vi "TDC_DAQV14_after_500MHz.vi"() -> ()   [LabVIEW 2017]
uses:
  <vilib>/Utility/file.llb/Write Delimited Spreadsheet (DBL).vi
  <vilib>/Utility/file.llb/Write Delimited Spreadsheet (I64).vi
panel:
  out "data out":string
  in  "display":bool
  in  "Thresholds":u16
  in  "one key for threshold":bool
  in  "save data":bool=TRUE
  in  "RST":bool
  out "rate":dbl=24091.155888084242
  in  "Thresholds (mV)":u16[](array[numeric])=[500, 500, 500, 500, 500, 500, 500, 500]
  out "appended path 2":path=path "G:/tdc/2017/test_20230331_123130.csv"
  in  "通道数量":i32=64
  out "Cal Table":u32[](array[numeric])=[100002, 100002, 100002, 100002, 100002, 100002, 100002, 100002, 100002, 100002, 100002, 100002, 100002, 100002, 100002, 100002, 100002, 100002, 100002, 100002, 100002, 100002, 100002, 100002, 100002, 100002, 100002, 100002, 100002, 100002, 100002, 100002, 100002, 100002, 100002, 100002, 100002, 100002, 100002, 100002, 100002, 100002, 100002, 100002, 100002, 100002, 100002, 100002, 100002, 100002, 100002, 100002, 100002, 100002, 100002, 100002, 100002, 100002, 100002, 100002, 100002, 100002, 100002, 100002]
  in  "channel for cal":i32=41
  out "single":u32 format="%08x"
  out "channel number":u64
  in  "bytes to read":i32=80
  out "Calibration Counter":i32=100000
  out "Event index":i32=97959
  out "cal":u32[](graph)=[0, 0, 0, 0, 0, 0, 0, 0, 0, 0, 0, 0, 0, 0, 0, 0, 0, 0, 0, 0, 0, 0, 0, 0, 0, 0, 0, 0, 0, 0, 0, 0, 0, 0, 0, 0, 0, 0, 0, 0, 0, 0, 0, 0, 0, 0, 0, 0, 0, 0, 0, 0, 0, 0, 0, 0, 0, 0, 0, 0, 0, 0, 0, 0, 0, 0, 0, 0, 0, 0, 0, 0, 0, 0, 0, 0, 0, 0, 0, 0, 0, 0, 0, 0, 0, 0, 0, 0, 0, 0, 0, 0, 0, 0, 0, 0, 0, 0, 0, 0, 0, 0, 0, 0, 0, 0, 0, 0, 0, 0, 0, 0, 0, 0, 0, 0, 0, 0, 0, 0, 0, 0, 0, 0, 0, 0, 0, 0, 0, 0, 0, 0, 0, 0, 0, 0, 0, 0, 0, 0, 0, 0, 0, 0, 0, 0, 0, 0, 0, 0, 0, 0, 0, 0, 0, 0, 0, 0, 0, 0, 0, 0, 0, 0, 0, 0, 0, 0, 0, 0, 0, 0, 0, 0, 0, 0, 0, 0, 0, 0, 0, 0, 0, 0, 0, 0, 0, 0, 0, 0, 0, 0, 0, 0, 0, 0, 0, 0, 0, 0, 0, 0, 0, 0, 0, 0, 0, 0, 0, 0, 0, 0, 0, 0, 0, 0, 0, 0, 0, 0, 0, 0, 0, 0, 0, 0, 0, 0, 0, 0, 0, 0, 0, 0, 0, 0, 0, 0, 0, 0, 0, 0, 0, 0, 0, 0, 0, 0, 0, 0, 0, 0, 0, 0, 0, 0, 0, 0, 0, 0, 0, 0, 0, 0, 0, 0, 0, 0, 0, 0, 0, 0, 0, 0, 0, 0, 0, 0, 0, 0, 0, 0, 0, 0, 69, 70, 200, 130, 69, 246, 200, 570, 155, 125, 160, 737, 265, 234, 80, 72, 155, 352, 178, 160, 101, 206, 84, 365, 186, 117, 86, 60, 156, 209, 124, 214, 202, 261, 117, 73, 308, 242, 175, 128, 73, 81, 167, 174, 75, 216, 363, 315, 84, 97, 67, 59, 109, 150, 167, 160, 255, 179, 72, 87, 290, 76, 119, 326, 114, 45, 62, 78, 150, 147, 151, 162, 202, 176, 82, 116, 138, 114, 75, 113, 110, 101, 122, 201, 217, 141, 136, 157, 107, 58, 72, 121, 214, 134, 190, 85, 127, 40, 49, 167, 84, 94, 55, 140, 150, 323, 144, 120, 198, 82, 104, 145, 98, 145, 124, 102, 120, 122, 116, 182, 125, 271, 123, 141, 162, 133, 69, 215, 207, 175, 168, 104, 108, 78, 53, 79, 151, 49, 89, 85, 85, 111, 122, 183, 115, 76, 52, 103, 55, 195, 80, 148, 66, 203, 83, 109, 86, 127, 131, 146, 160, 56, 237, 116, 94, 113, 99, 196, 68, 98, 110, 100, 172, 79, 169, 116, 117, 123, 110, 65, 74, 191, 201, 60, 82, 145, 203, 331, 56, 81, 133, 70, 159, 77, 112, 99, 387, 124, 150, 144, 130, 139, 195, 199, 128, 218, 147, 185, 205, 192, 146, 108, 97, 131, 101, 111, 84, 118, 163, 85, 177, 88, 182, 180, 61, 157, 82, 351, 115, 106, 74, 143, 109, 258, 313, 81, 165, 89, 58, 85, 204, 137, 246, 384, 77, 54, 56, 35, 35, 56, 80, 104, 166, 240, 104, 141, 174, 99, 41, 45, 48, 342, 180, 52, 34, 51, 82, 107, 274, 80, 228, 263, 129, 87, 73, 132, 104, 176, 471, 227, 175, 92, 123, 87, 132, 208, 250, 311, 62, 78, 114, 117, 138, 66, 205, 68, 65, 77, 89, 222, 101, 35, 32, 93, 426, 159, 207, 108, 118, 397, 204, 160, 183, 94, 81, 319, 221, 353, 107, 148, 53, 77, 134, 155, 112, 111, 231, 165, 106, 57, 49, 105, 122, 283, 91, 135, 227, 130, 44, 139, 101, 136, 222, 141, 96, 146, 191, 123, 61, 106, 123, 177, 186, 188, 104, 123, 156, 140, 100, 64, 374, 103, 60, 168, 144, 148, 130, 95, 162, 194, 107, 167, 74, 45, 67, 215, 229, 107, 63, 222, 202, 123, 240, 160, 148, 120, 139, 175, 82, 103, 141, 143, 202, 174, 62, 150, 156, 284, 140, 86, 136, 150, 198, 220, 264, 88, 56, 69, 65, 69, 85, 66, 84, 107, 133, 510, 177, 52, 53, 55, 110, 95, 96, 83, 124, 150, 123, 178, 95, 62, 75, 88, 69, 95, 35, 50, 75, 183, 97, 251, 162, 179, 180, 93, 65, 169, 112, 116, 177, 208, 184, 68, 75, 142, 98, 71, 150, 172, 202, 395, 214, 117, 49, 50, 82, 91, 115, 199, 198, 93, 89, 64, 109, 107, 126, 100, 146, 150, 289, 93, 85, 109, 265, 257, 120, 105, 81, 143, 123, 142, 119, 95, 119, 215, 82, 168, 280, 111, 80, 82, 356, 76, 69, 92, 169, 83, 86, 299, 88, 276, 65, 78, 63, 82, 83, 177, 100, 201, 200, 190, 121, 241, 193, 119, 52, 71, 41, 83, 299, 57, 49, 89, 383, 57, 104, 116, 97, 125, 140, 90, 500, 118, 131, 99, 266, 88, 120, 136, 137, 67, 284, 70, 104, 197, 134, 97, 65, 58, 91, 59, 60, 151, 249, 196, 119, 123, 237, 171, 123, 194, 186, 327, 72, 73, 99, 109, 71, 77, 83, 280, 299, 156, 122, 105, 70, 71, 57, 69, 134, 243, 113, 44, 98, 115, 59, 69, 95, 101, 71, 91, 99, 174, 162, 58, 64, 63, 516, 81, 69, 57, 41, 74, 56, 81, 52, 102, 98, 117, 102, 214, 291, 137, 66, 67, 101, 69, 93, 95, 166, 66, 117, 262, 138, 91, 82, 112, 120, 164, 98, 141, 218, 129, 81, 149, 194, 418, 79, 63, 79, 143, 157, 171, 123, 164, 295, 81, 83, 71, 229, 94, 291, 240, 117, 169, 63, 155, 82, 115, 184, 82, 120, 90, 124, 256, 88, 117, 146, 38, 47, 368, 150, 86, 26, 89, 131, 94, 175, 84, 175, 206, 184, 110, 89, 134, 125, 258, 82, 248, 85, 82, 183, 85, 284, 160, 108, 55, 60, 137, 59, 58, 105, 136, 68, 51, 58, 290, 461, 126, 83, 52, 150, 63, 27, 40, 19, 10, 2, 0, 0, 0, 0, 0, 0, 0, 0, 0, 0, 0, 0, 0, 0, 0, 0, 0, 0, 0, 0, 0, 0, 0, 0, 0, 0, 0, 0, 0, 0, 0, 0, 0, 0, 0, 0, 0, 0, 0, 0, 0, 0, 0, 0, 0, 0, 0, 0, 0, 0, 0, 0, 0, 0, 0, 0, 0, 0, 0, 0, 0, 0, 0, 0, 0, 0, 0, 0, 0, 0, 0, 0, 0, 0, 0, 0, 0, 0, 0, 0, 0, 0, 0, 0, 0, 0, 0, 0, 0, 0, 0, 0, 0, 0, 0, 0, 0, 0, 0, 0, 0, 0, 0, 0, 0, 0, 0, 0, 0, 0, 0, 0, 0, 0, 0, 0, 0, 0, 0, 0, 0, 0, 0, 0, 0, 0, 0, 0, 0, 0, 0, 0, 0, 0, 0, 0, 0, 0, 0, 0, 0, 0, 0, 0, 0, 0, 0, 0, 0, 0, 0, 0, 0, 0, 0, 0, 0, 0, 0, 0, 0, 0, 0, 0, 0, 0, 0, 0, 0, 0, 0, 0, 0, 0, 0, 0, 0, 0, 0, 0, 0, 0, 0, 0, 0, 0, 0, 0, 0, 0, 0, 0, 0, 0, 0, 0, 0, 0, 0, 0, 0, 0, 0, 0, 0, 0, 0, 0, 0, 0, 0, 0, 0, 0, 0, 0, 0, 0, 0, 0, 0, 0, 0, 0, 0, 0, 0, 0, 0, 0, 0, 0, 0, 0, 0, 0, 0, 0, 0, 0, 0, 0, 0, 0, 0, 0, 0, 0, 0, 0, 0, 0, 0, 0, 0, 0, 0, 0, 0, 0, 0, 0, 0, 0, 0, 0, 0, 0, 0, 0, 0, 0, 0, 0, 0, 0, 0, 0, 0, 0, 0, 0, 0, 0, 0, 0, 0, 0, 0, 0, 0, 0, 0, 0, 0, 0, 0, 0, 0, 0, 0, 0, 0, 0, 0, 0, 0, 0, 0, 0, 0, 0, 0, 0, 0, 0, 0, 0, 0, 0, 0, 0, 0, 0, 0, 0, 0, 0, 0, 0, 0, 0, 0, 0, 0, 0, 0, 0, 0, 0, 0, 0, 0, 0, 0, 0, 0, 0, 0, 0, 0, 0, 0, 0, 0, 0, 0, 0, 0, 0, 0, 0, 0, 0, 0, 0, 0, 0, 0, 0, 0, 0, 0, 0, 0, 0, 0, 0, 0, 0, 0, 0, 0, 0, 0, 0, 0, 0, 0, 0, 0, 0, 0, 0, 0, 0, 0, 0, 0, 0, 0, 0, 0, 0, 0, 0, 0, 0, 0, 0, 0, 0, 0, 0, 0, 0, 0, 0, 0, 0, 0, 0, 0, 0, 0, 0, 0, 0, 0, 0, 0, 0, 0, 0, 0, 0, 0, 0, 0, 0, 0, 0, 0, 0, 0, 0, 0, 0, 0, 0, 0, 0, 0, 0, 0, 0, 0, 0, 0, 0, 0, 0, 0, 0, 0, 0, 0, 0, 0, 0, 0, 0, 0, 0, 0, 0, 0, 0, 0, 0, 0, 0, 0, 0, 0, 0, 0, 0, 0, 0, 0, 0, 0, 0, 0, 0, 0, 0, 0, 0, 0, 0, 0, 0, 0, 0, 0, 0, 0, 0, 0, 0, 0, 0, 0, 0, 0, 0, 0, 0, 0, 0, 0, 0, 0, 0, 0, 0, 0, 0, 0, 0, 0, 0, 0, 0, 0, 0, 0, 0, 0, 0, 0, 0, 0, 0, 0, 0, 0, 0, 0, 0, 0, 0, 0, 0, 0, 0, 0, 0, 0, 0, 0, 0, 0, 0, 0, 0, 0, 0, 0, 0, 0, 0, 0, 0, 0, 0, 0, 0, 0, 0, 0, 0, 0, 0, 0, 0, 0, 0, 0, 0, 0, 0, 0, 0, 0, 0, 0, 0, 0, 0, 0, 0, 0, 0, 0, 0, 0, 0, 0, 0, 0, 0, 0, 0, 0, 0, 0, 0, 0, 0, 0, 0, 0, 0, 0, 0, 0, 0, 0, 0, 0, 0, 0, 0, 0, 0, 0, 0, 0, 0, 0, 0, 0, 0, 0, 0, 0, 0, 0, 0, 0, 0, 0, 0, 0, 0, 0, 0, 0, 0, 0, 0, 0, 0, 0, 0, 0, 0, 0, 0, 0, 0, 0, 0, 0, 0, 0, 0, 0, 0, 0, 0, 0, 0, 0, 0, 0, 0, 0, 0, 0, 0, 0, 0, 0, 0, 0, 0, 0, 0, 0, 0, 0, 0, 0, 0, 0, 0, 0, 0, 0, 0, 0, 0, 0, 0, 0, 0, 0, 0, 0, 0, 0, 0, 0, 0, 0, 0, 0, 0, 0, 0, 0, 0, 0, 0, 0, 0, 0, 0, 0, 0, 0, 0, 0, 0, 0, 0, 0, 0, 0, 0, 0, 0, 0, 0, 0, 0, 0, 0, 0, 0, 0, 0, 0, 0, 0, 0, 0, 0, 0, 0, 0, 0, 0, 0, 0, 0, 0, 0, 0, 0, 0, 0, 0, 0, 0, 0, 0, 0, 0, 0, 0, 0, 0, 0, 0, 0, 0, 0, 0, 0, 0, 0, 0, 0, 0, 0, 0, 0, 0, 0, 0, 0, 0, 0, 0, 0, 0, 0, 0, 0, 0, 0, 0, 0, 0, 0, 0, 0, 0, 0, 0, 0, 0, 0, 0, 0, 0, 0, 0, 0, 0, 0, 0, 0, 0, 0, 0, 0, 0, 0, 0, 0, 0, 0, 0, 0, 0, 0, 0, 0, 0, 0, 0, 0, 0, 0, 0, 0, 0, 0, 0, 0, 0, 0, 0, 0, 0, 0, 0, 0, 0, 0, 0, 0, 0, 0, 0, 0, 0, 0, 0, 0, 0, 0, 0, 0, 0, 0, 0, 0, 0, 0, 0, 0, 0, 0, 0, 0, 0, 0, 0, 0, 0, 0, 0, 0, 0, 0, 0, 0, 0, 0, 0, 0, 0, 0, 0, 0, 0, 0, 0, 0, 0, 0, 0, 0, 0, 0, 0, 0, 0, 0, 0, 0, 0, 0, 0, 0, 0, 0, 0, 0, 0, 0, 0, 0, 0, 0, 0, 0, 0, 0, 0, 0, 0, 0, 0, 0, 0, 0, 0, 0, 0, 0, 0, 0, 0, 0, 0, 0, 0, 0, 0, 0, 0, 0, 0, 0, 0, 0, 0, 0, 0, 0, 0, 0, 0, 0, 0, 0, 0, 0, 0, 0, 0, 0, 0, 0, 0, 0, 0, 0, 0, 0, 0, 0, 0, 0, 0, 0, 0, 0, 0, 0, 0, 0, 0, 0, 0, 0, 0, 0, 0]
  out "error out":errorcluster
  in  "stop":bool=TRUE
  out "appended path":path=path "G:/tdc/2017/test_20230331_123130.dat"
  in  "filename":string="test"
  in  "Events":i32=110000 min=1
  in  "timeout (ms)":i32=10000
  in  "address":string="192.168.10.10"
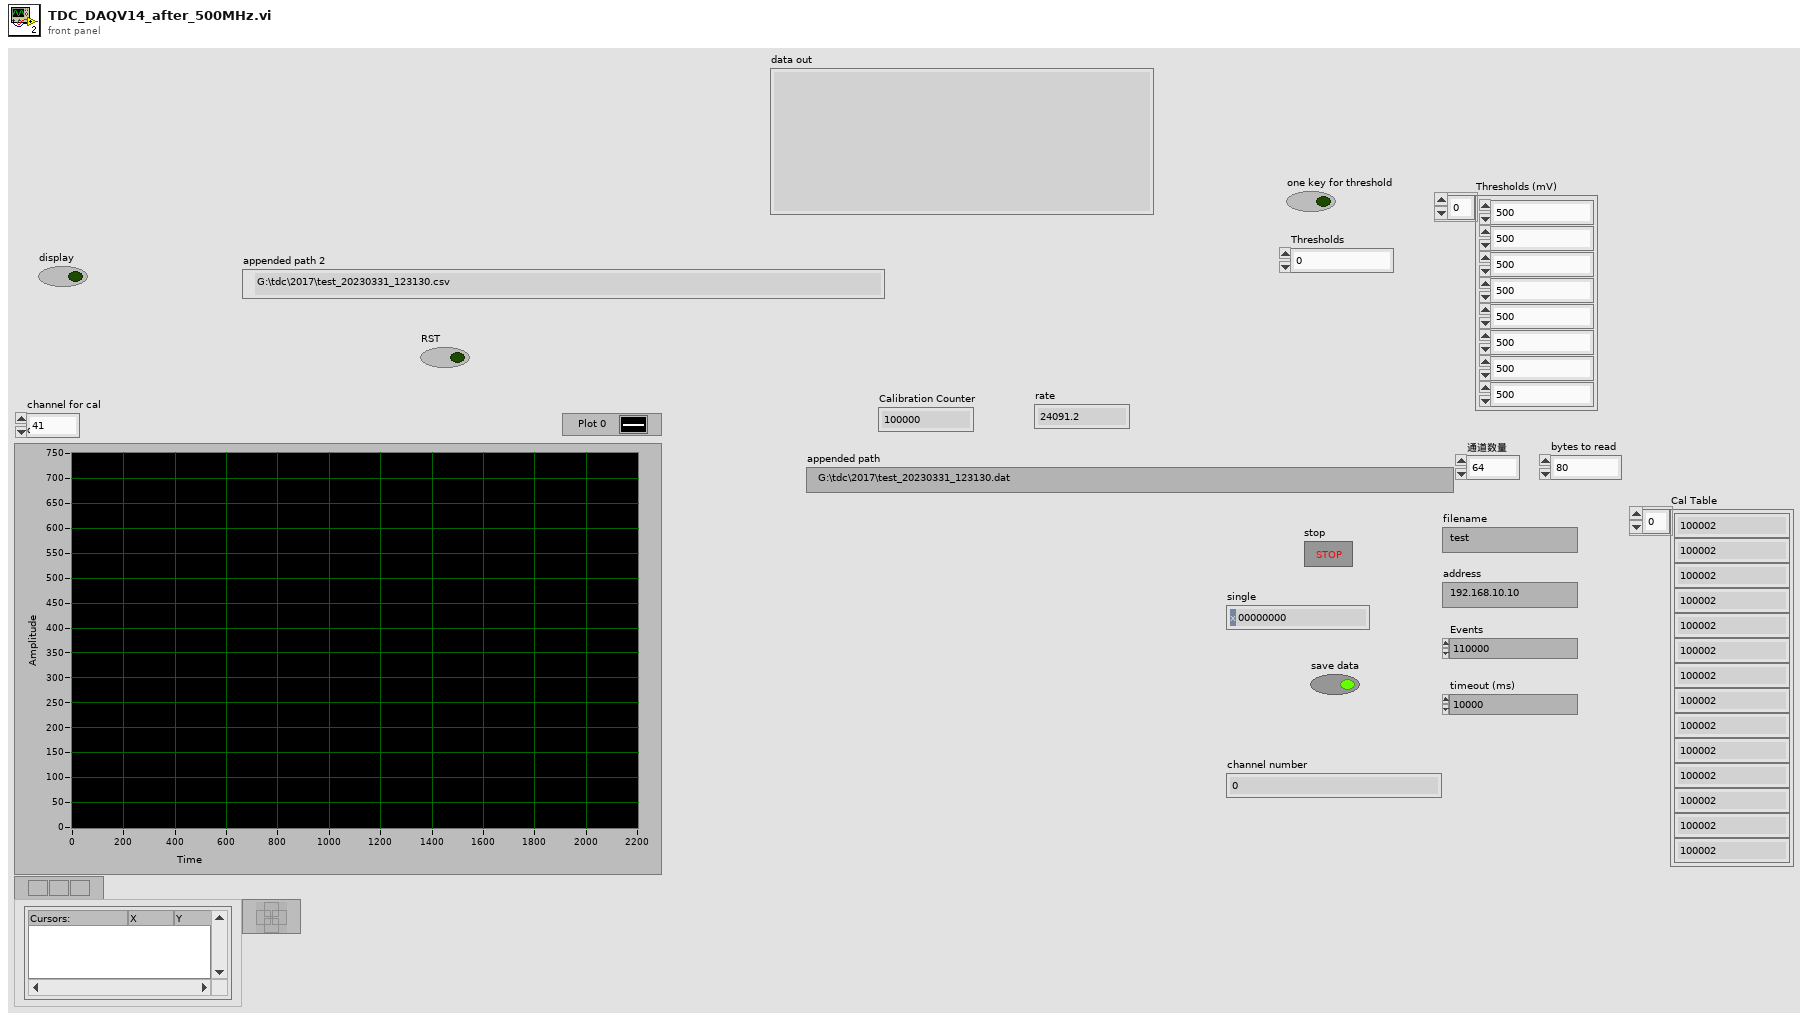
[diagram p1: front panel]
types:
  T1 = enum16{"open", "replace", "create", "open or create", "replace or create", "replace or create with confirmation"}
  T2 = enum16{"big-endian, network order", "native, host order", "little-endian"}
  T3 = enum16{"Standard", "Buffered", "CRLF", "Immediate"}
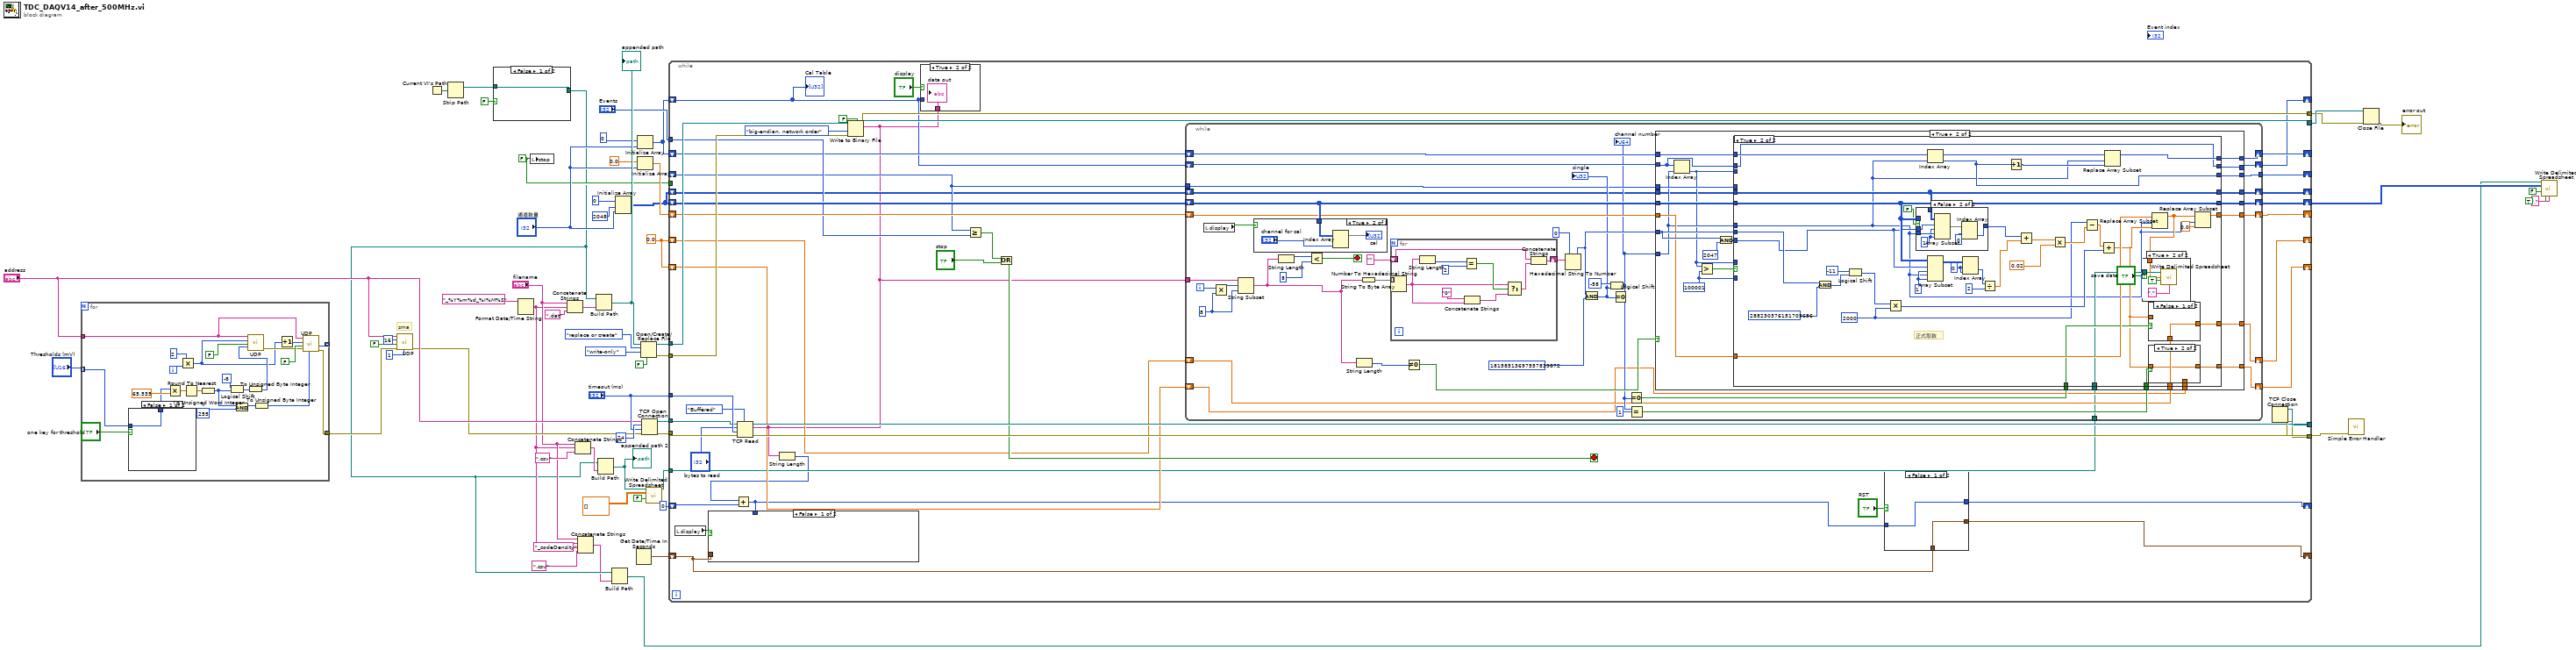
[diagram p0: block diagram]
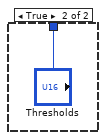
[diagram p2: hidden frame]
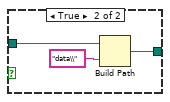
[diagram p3: hidden frame]
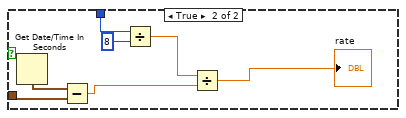
[diagram p4: hidden frame]
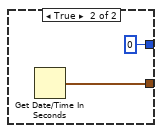
[diagram p6: hidden frame]
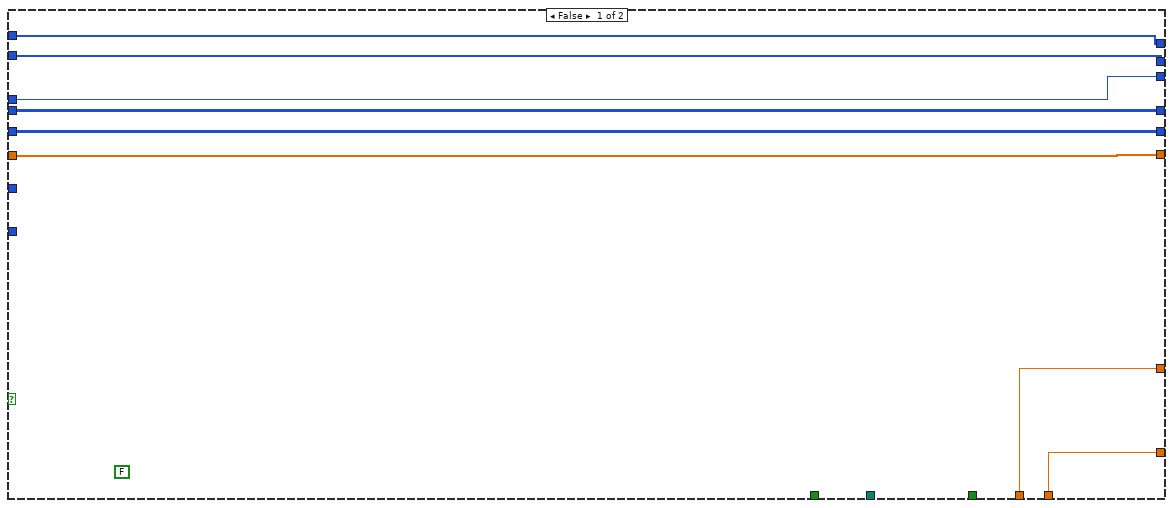
[diagram p8: hidden frame]
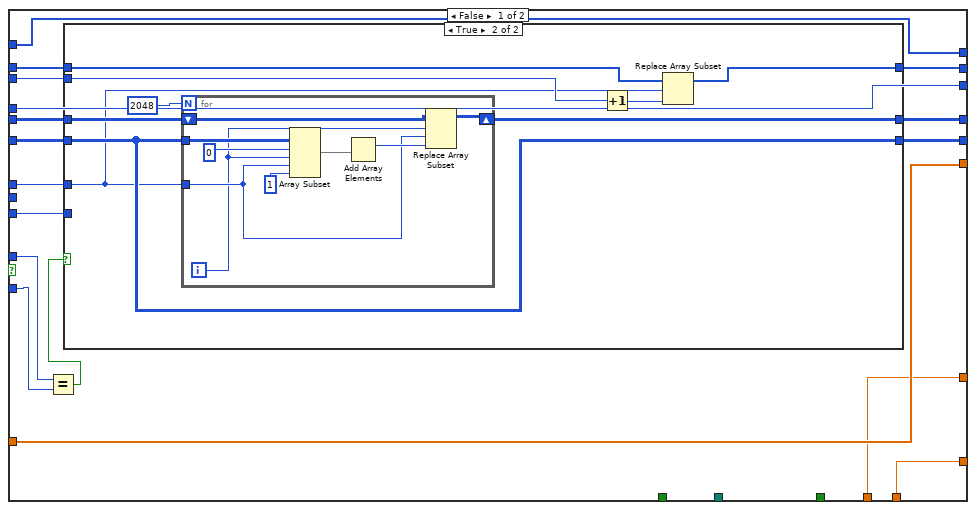
[diagram p9: hidden frame]
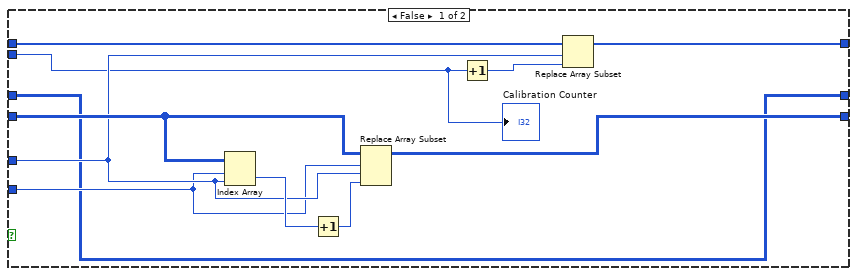
[diagram p10: hidden frame]
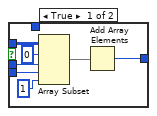
[diagram p12: hidden frame]
diagram:
  w12 = FALSE ("stop")
  w29 = 0.0
  # "sma"
  n1 = for {
    tunnel: "address" -> [w76]
    tunnel: "Thresholds (mV)" -> [w60] mode=indexing
    tunnel: [w69] -> _ mode=indexing
    tunnel: [w63] -> w16
    i -> [w82]
    w71 = u16 255  # x
    n2 = case shown="False" "one key for threshold" {
      tunnel: [w83 "Thresholds"] -> w61
      tunnel: w60 -> [w83 _]
      frame False {
      }
      frame True {
      }
    }
    n3 = Multiply(x=w61, y=65.535) -> (x*y=w79:dbl)
    n4 = Multiply(x=2, y=w82) -> (x*y=w64:i32)
    n5 = Round To Nearest(number=w79) -> (nearest integer value=w77:dbl)
    n6 = To Unsigned Word Integer(number=w77) -> (unsigned 16bit integer=w66:u16)
    n7 = Logical Shift(y=i16 -8, x=w66) -> (x << y=w73:u16)
    n8 = And(x=w66, y=w71) -> (x .and. y?=w70:u16)
    n9 = To Unsigned Byte Integer(number=w73) -> (unsigned 8bit integer=w72:u8)
    n10 = call "UDP.vi"("In"=w72, "Read (TRUE)"=FALSE, "Address"=w64, "IP address"=w76) -> ("error out"=w65:errorcluster)  [unwired: 5 in, 1 out]
    n11 = To Unsigned Byte Integer(number=w70) -> (unsigned 8bit integer=w68:u8)
    n12 = Increment(x=w64) -> (x+1=w75:i32)
    n13 = call "UDP.vi"("In"=w68, "error in (no error)"=w65, "Read (TRUE)"=FALSE, "Address"=w75, "IP address"=w76) -> ("error out"=w63:errorcluster, "Out"=w69:u8)  [unwired: 4 in]
  }
  n14 = call "UDP.vi"("In"=u8 1, "error in (no error)"=w16, "Read (TRUE)"=FALSE, "Address"=u32 16, "IP address"="address") -> ("error out"=w15:errorcluster)  [unwired: 4 in, 1 out]
  n15 = Current VI's Path() -> (path=w49:path)
  n16 = Strip Path(path=w49) -> (stripped path=w48:path)  [unwired: 1 out]
  n17 = case shown="False" FALSE {
    tunnel: w48 -> [w85 w87]
    tunnel: [w85 w86] -> w7
    frame False {
    }
    frame True {
      n18 = Build Path(base path=w87, name or relative path="data\\") -> (appended path=w86:path)
    }
  }
  n19 = Format Date/Time String(time format string (%c)="_%Y%m%d_%I%M%S") -> (date/time string=w10:string)  [unwired: 2 in]
  n20 = local write "stop"(w12) -> ()
  n21 = Concatenate Strings("filename", w10, ".dat") -> (w47:string)
  n22 = Concatenate Strings("filename", w10, ".csv") -> (w31:string)
  n23 = Concatenate Strings("filename", w10, "_codeDensity" ("string"), ".csv") -> (w6:string)
  n24 = Build Path(base path=w7, name or relative path=w47) -> (appended path=w46:path)
  "appended path" <- w46
  n25 = Build Path(base path=w7, name or relative path=w31) -> (appended path=w26:path)
  "appended path 2" <- w26
  n26 = Build Path(base path=w7, name or relative path=w6) -> (appended path=w3:path)
  n27 = Initialize Array(u32 0 ("element"), 2048 ("dimension size"), "通道数量") -> (w28:u32[][])
  n28 = Get Date/Time In Seconds() -> (seconds since 1Jan1904=w19:timestamp)
  n29 = Initialize Array(u32 0 ("element"), "通道数量") -> (w30:u32[])
  n30 = Initialize Array(0.0, "通道数量") -> (w36:dbl[])
  n31 = Open/Create/Replace File(file path (use dialog)=w46, operation (0:open)=T1."replace or create", access (0:read/write)=enum16{"read/write", "read-only", "write-only"}."write-only", disable buffering (F)=FALSE) -> (refnum out=w51:refnum<file>, error out=w50:errorcluster)  [unwired: 2 in, 1 out]
  n32 = TCP Open Connection(address="address", remote port or service name=u16 24 ("port"), timeout ms (60000)="timeout (ms)", error in (no error)=w15) -> (connection ID=w56:refnum<k5>, error out=w55:errorcluster)  [unwired: 1 in]
  n33 = call-poly <vilib>:"Write Delimited Spreadsheet.vi"("file path (dialog if empty)"=w26, "2D data"=dbl[][] [], "append to file? (new file:F)"=FALSE) -> ("new file path (Not A Path if cancelled)"=w25:path)  [unwired: 11 in, 1 out]
  n34 = while {
    tunnel: "timeout (ms)" -> [w132]
    tunnel: w56 -> [w131]
    tunnel: w55 -> [w130]
    tunnel: w51 -> [w125]
    tunnel: w50 -> [w126]
    tunnel: [w128] -> w43
    tunnel: [w127] -> w42
    tunnel: [w124] -> w41
    tunnel: [w123] -> w40
    shift-right: [w119] -> w4
    shift-left: w28 -> [w120]
    shift-right: [w102] -> _
    shift-left: w36 -> [w118]
    tunnel: "Events" -> [w114]
    shift-right: [w113] -> _
    shift-left: w30 -> [w112]
    shift-right: [w111] -> _
    shift-left: _ -> [w110]
    shift-right: [w109] -> _
    shift-left: w30 -> [w90]
    shift-right: [w108] -> _
    shift-left: w29 -> [w105]
    shift-right: [w107] -> _
    shift-left: w29 -> [w106]
    shift-right: [w93] -> _
    shift-left: w28 -> [w104]
    tunnel: w25 -> [w103]
    shift-right: [w97] -> _
    shift-left: 0 -> [w101]
    shift-right: [w95] -> _
    shift-left: w19 -> [w94]
    tunnel: w12 -> [_]
    stop <- w117 stop-if-true
    n35 = local read "display"() -> (w91:bool)
    n36 = TCP Read(connection ID=w131, bytes to read="bytes to read", error in (no error)=w130, 7:T3."Buffered" ("mode (standard)"), 9:w132) -> (connection ID out=w128:refnum<k5>, data out=w89:string, error out=w127:errorcluster)
    n37 = String Length(string=w89) -> (length=w99:i32)
    n38 = Add(x=w99, y=w101) -> (x+y=w98:i32)
    n39 = case shown="False" w91 {
      tunnel: w98 -> [_ w134]
      tunnel: w94 -> [_ w133]
      frame False {
      }
      frame True {
        n40 = Get Date/Time In Seconds() -> (seconds since 1Jan1904=w138:timestamp)
        n41 = Subtract(x=w138, y=w133) -> (x-y=w137:dbl)
        n42 = Divide(x=w134, y=8) -> (x/y=w136:dbl)
        n43 = Divide(x=w136, y=w137) -> (x/y=→"rate":dbl)
      }
    }
    n44 = Write to Binary File(file (use dialog)=w125, data=w89, error in=w126, 5:FALSE ("prepend array or string size? (T)"), 9:T2."big-endian, network order" ("byte order (0:big-endian, network order)")) -> (refnum out=w124:refnum<file>, error out=w123:errorcluster)  [unwired: 1 in, 1 out]
    n45 = case shown="True" "display" {
      tunnel: w90 -> [_ _]
      tunnel: w89 -> [_ w140]
      frame False {
      }
      frame True {
        "data out" <- w140
      }
    }
    n46 = Greater Or Equal?(x=w110, y=w114) -> (x >= y?=w115:bool)
    n47 = Or(x=w115, y="stop") -> (x .or. y?=w117:bool)
    n48 = while {
      tunnel: w89 -> [w180]
      shift-right: [w176] -> w119
      shift-left: w120 -> [w174]
      shift-right: [w172] -> w102
      shift-left: w118 -> [w173]
      shift-right: [w166] -> w113
      shift-left: w112 -> [w165]
      tunnel: [w164] -> w111
      tunnel: w110 -> [w163]
      shift-right: [w161] -> w109
      shift-left: w90 -> [w162]
      shift-right: [w153] -> w108
      shift-left: w105 -> [w151]
      shift-right: [w149] -> w107
      shift-left: w106 -> [w150]
      tunnel: w103 -> [w147]
      shift-right: [w146] -> w93
      shift-left: w104 -> [w148]
      i -> [w178]
      stop <- w169 stop-if-true
      w177 = 8 ("length (rest)")
      n49 = local read "display"() -> (w145:bool)
      n50 = Multiply(x=w178, y=w177) -> (x*y=w179:i32)
      n51 = String Subset(string=w180, offset (0)=w179, length (rest)=w177) -> (substring=w160:string)
      n52 = case shown="True" w145 {
        tunnel: w174 -> [_ w187]
        frame False {
        }
        frame True {
          n53 = Index Array(array=w187, index (col)="channel for cal") -> (element=→"cal":u32[])  [unwired: 1 in]
        }
      }
      n54 = String Length(string=w160) -> (length=w171:i32)
      n55 = Less?(x=w171, y=8) -> (x < y?=w169:bool)
      n56 = String Length(string=w160) -> (length=w158:i32)
      n57 = String To Byte Array(string=w160) -> (unsigned byte array=w183:u8[])
      n58 = for {
        shift-right: [w339] -> w182
        shift-left: "" ("format string") -> [w336]
        tunnel: w183 -> [w340] mode=indexing
        n59 = Number To Hexadecimal String(2:w340) -> (0:w332:string)  [unwired: 1 in]
        n60 = String Length(string=w332) -> (length=w338:i32)
        n61 = Equal?(x=w338, y=2) -> (x = y?=w335:bool)
        n62 = Concatenate Strings("0" ("format string"), w332) -> (w334:string)
        n63 = Select(t=w332, s=w335, f=w334) -> (s? t:f=w331:string)
        n64 = Concatenate Strings(w336, w331) -> (w339:string)
      }
      n65 = Not Equal To 0?(x=w158) -> (x != 0?=w157:bool)
      n66 = Hexadecimal String To Number(string=w182, default (0uL)=u64 0 ("default (0 U32)")) -> (number=w175:u64)  [unwired: 1 in, 1 out]
      n67 = And(x=w175, y=u64 18158513697557839872 ("port")) -> (x .and. y?=w167:u64)
      "single" <- w167
      n68 = Logical Shift(y=i16 -58, x=w167) -> (x << y=w156:u64)
      "channel number" <- w156
      n69 = Equal To 0?(x=w167) -> ()  [unwired: 1 out]
      n70 = Equal To 0?(x=w156) -> (x = 0?=w154:bool)
      n71 = Equal?(x=w156, y=u64 1) -> (x = y?=w152:bool)
      n72 = case shown="True" w157 {
        tunnel: w175 -> [_ w221]
        tunnel: w163 -> [w192 w211]
        tunnel: w174 -> [w195 w220]
        tunnel: [w195 w219] -> w176
        tunnel: [w194 w216] -> w172
        tunnel: w173 -> [w194 w215]
        tunnel: w156 -> [_ w210]
        tunnel: w165 -> [w193 w214]
        tunnel: [w193 w213] -> w166
        tunnel: [w192 w212] -> w164
        tunnel: w162 -> [w191 w209]
        tunnel: [w191 w208] -> w161
        tunnel: w154 -> [_ w207]
        tunnel: w151 -> [w190 w206]
        tunnel: [w190 w205] -> w153
        tunnel: w152 -> [_ w204]
        tunnel: w150 -> [w189 w203]
        tunnel: [w189 w202] -> w149
        tunnel: w148 -> [w188 w199]
        tunnel: [w188 w198] -> w146
        tunnel: w147 -> [_ w197]
        frame False {
          (unwired) FALSE
        }
        frame True {
          w200 = 100001 ("y")
          n73 = Index Array(array=w209, index=w210) -> (element=w201:u32)
          n74 = Greater?(x=w201, y=w200) -> (0:w196:bool)
          n75 = And(x=w221, y=u64 2047 ("port")) -> (x .and. y?=w217:u64)
          n76 = case shown="True" w196 {
            tunnel: w221 -> [_ w308]
            tunnel: w220 -> [w238 w291]
            tunnel: [w237 w291] -> w219
            tunnel: w217 -> [w229 w289]
            tunnel: [w236 w273] -> w216
            tunnel: w215 -> [w236 w298]
            tunnel: w211 -> [w234 _]
            tunnel: w210 -> [w232 w271]
            tunnel: w214 -> [w235 w297]
            tunnel: [w235 w296] -> w213
            tunnel: [w234 w294] -> w212
            tunnel: w201 -> [w230 _]
            tunnel: w209 -> [w233 w293]
            tunnel: [w231 w293] -> w208
            tunnel: w207 -> [_ w285]
            tunnel: w206 -> [w228 w284]
            tunnel: [w228 w283] -> w205
            tunnel: w204 -> [_ w282]
            tunnel: w203 -> [w227 w281]
            tunnel: [w227 w280] -> w202
            tunnel: w201 -> [w225 _]
            tunnel: w200 -> [w222 _]
            tunnel: w199 -> [w224 w275]
            tunnel: [w223 w275] -> w198
            tunnel: w197 -> [_ w274]
            frame False {
              n77 = Equal?(x=w225, y=w222) -> (x = y?=w226:bool)
              n78 = case shown="True" w226 {
                tunnel: w238 -> [w249 w255]
                tunnel: [w247 w255] -> w237
                tunnel: w233 -> [w245 w253]
                tunnel: w232 -> [w244 w250]
                tunnel: [w242 w252] -> w231
                tunnel: w230 -> [w241 w251]
                tunnel: w229 -> [w240 _]
                tunnel: w224 -> [w239 w257]
                tunnel: [w239 w256] -> w223
                frame False {
                  n79 = Index Array(array=w249, index (row)=w240, index (col)=w244) -> (element=w248:u32)
                  n80 = Increment(x=w248) -> (x+1=w246:u32)
                  n81 = Replace Array Subset(array=w249, new element=w246, index (row)=w240, index (col)=w244) -> (w247:u32[][])
                  n82 = Increment(x=w241) -> (x+1=w243:u32)
                  n83 = Replace Array Subset(array=w245, new element=w243, index=w244) -> (w242:u32[])
                  "Calibration Counter" <- w241
                }
                frame True {
                  n84 = for {
                    N: 2048 -> [_]
                    tunnel: w255 -> [w267]
                    tunnel: w250 -> [w260]
                    shift-right: [w262] -> w256
                    shift-left: w257 -> [w263]
                    i -> [w259]
                    n85 = Array Subset(array=w267, index (row)=0 ("索引"), length (row)=w259, index (col)=w260, length (col)=1 ("长度")) -> (w264:u32[][])
                    n86 = Add Array Elements(numeric array=w264) -> (sum=w261:u32)
                    n87 = Replace Array Subset(array=w263, new element=w261, index (row)=w259, index (col)=w260) -> (w262:u32[][])
                  }
                  n88 = Increment(x=w251) -> (x+1=w254:u32)
                  n89 = Replace Array Subset(array=w253, new element=w254, index=w250) -> (w252:u32[])
                }
              }
            }
            frame True {
              w287 = 0 ("索引 (行)")
              w290 = 1 ("长度")
              w268 = u64 2000 ("y")
              # "正式取数"
              n90 = And(x=w308, y=u64 288230376151709696 ("port")) -> (x .and. y?=w305:u64)
              n91 = Logical Shift(y=i16 -11, x=w305) -> (x << y=w300:u64)
              n92 = Multiply(x=w300, y=w268) -> (x*y=w299:u64)
              n93 = case shown="False" FALSE {
                tunnel: [w314 w321] -> w303
                tunnel: w291 -> [w317 _]
                tunnel: w271 -> [w316 w326]
                tunnel: w289 -> [w315 w324]
                tunnel: w275 -> [_ w325]
                frame True {
                  n94 = Array Subset(array=w317, index (row)=0 ("索引"), length (row)=w315, index (col)=w316, length (col)=1 ("长度")) -> (w318:u32[][])
                  n95 = Add Array Elements(numeric array=w318) -> (sum=w314:u32)
                }
                frame False {
                  w320 = 0 ("index (row)")
                  w323 = 1 ("长度")
                  n96 = Array Subset(array=w325, index (row)=w324, length (row)=w323, index (col)=w326, length (col)=w323) -> (w322:u32[][])
                  n97 = Index Array(array=w322, index (row)=w320, index (col)=w320) -> (element=w321:u32)
                }
              }
              n98 = Index Array(array=w297, index=w271) -> (element=w294:u32)
              n99 = Array Subset(array=w291, index (row)=w289, length (row)=w290, index (col)=w271, length (col)=w290) -> (w288:u32[][])
              n100 = Index Array(array=w288, index (row)=w287, index (col)=w287) -> (element=w286:u32)
              n101 = Divide(x=w286, y=u32 2) -> (x/y=w292:dbl)
              n102 = Increment(x=w294) -> (x+1=w295:u32)
              n103 = Add(x=w303, y=w292) -> (x+y=w302:dbl)
              n104 = Multiply(x=w302, y=0.02) -> (x*y=w278:dbl)
              n105 = Subtract(x=w268, y=w278) -> (x-y=w277:dbl)
              n106 = Add(x=w277, y=w299) -> (x+y=w279:dbl)
              n107 = Replace Array Subset(array=w297, new element=w295, index=w271) -> (w296:u32[])
              n108 = case shown="False" w285 {
                tunnel: w279 -> [_ w330]
                tunnel: [w329 w330] -> w283
                tunnel: w284 -> [w329 _]
                frame False {
                }
                frame True {
                }
              }
              n109 = case shown="True" w282 {
                tunnel: [w327 w328] -> w280
                tunnel: w281 -> [w327 _]
                tunnel: w279 -> [_ w328]
                frame False {
                }
                frame True {
                }
              }
              n110 = Replace Array Subset(array=w298, new element=w279, index=w271) -> (w272:dbl[])
              n111 = case shown="True" "save data" {
                tunnel: w274 -> [_ w312]
                tunnel: w272 -> [_ w309]
                frame False {
                }
                frame True {
                  n112 = call-poly <vilib>:"Write Delimited Spreadsheet.vi"("file path (dialog if empty)"=w312, "1D data"=w309, "append to file? (new file:F)"=TRUE, "delimiter (\\t)"="," ("delimiter (\\t)")) -> ()  [unwired: 10 in, 2 out]
                }
              }
              n113 = Replace Array Subset(array=w272, new element=0.0 ("new element/subarray"), index=w271) -> (w273:dbl[])
            }
          }
        }
      }
    }
    n114 = case shown="False" "RST" {
      tunnel: w98 -> [w142 _]
      tunnel: [w142 0] -> w97
      tunnel: [w141 w143] -> w95
      tunnel: w94 -> [w141 _]
      frame False {
      }
      frame True {
        n115 = Get Date/Time In Seconds() -> (seconds since 1Jan1904=w143:timestamp)
      }
    }
    "Cal Table" <- w90
  }
  n116 = TCP Close Connection(connection ID=w43, error in (no error)=w42) -> (error out=w58:errorcluster)  [unwired: 1 in, 1 out]
  n117 = call <vilib>:"Simple Error Handler.vi"("error in (no error)"=w58) -> ()  [unwired: 4 in, 5 out]
  n118 = Close File(refnum=w41, error in=w40) -> (error out=→"error out":errorcluster)  [unwired: 1 out]
  n119 = call-poly <vilib>:"Write Delimited Spreadsheet.vi"("file path (dialog if empty)"=w3, "2D data"=w4, "append to file? (new file:F)"=FALSE, "transpose? (no:F)"=TRUE, "delimiter (\\t)"="," ("delimiter (\\t)")) -> ()  [unwired: 9 in, 2 out]
